vi "Apply special move.vi"(8 "error in (no error)":errorcluster, 10 "Position in":refnum<class "Position.lvclass">, 11 "DoublePush in":refnum<class "DoublePush.lvclass">) -> (0 "error out":errorcluster, 2 "Position out":refnum<class "Position.lvclass">, 3 "DoublePush out":refnum<class "DoublePush.lvclass">)   [LabVIEW 2015, in "Chesslib.lvlib" / "DoublePush.lvclass"]
uses:
  DoublePush.lvclass
  Position/Position.lvclass
  DoublePush.lvclass/DoublePush.ctl
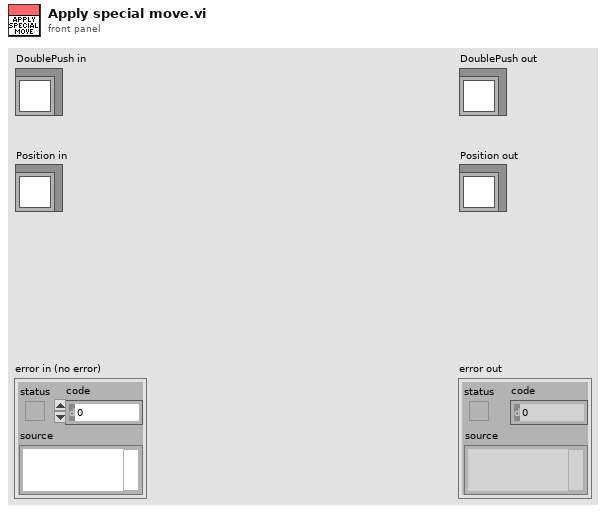
[diagram p1: front panel]
types:
  T1 = typedef "Chesslib.lvlib/Square.ctl" = cluster{"File":T2, "Rank":T3}
  T2 = typedef "Chesslib.lvlib/File.ctl" = enum8{"a", "b", "c", "d", "e", "f", "g", "h"}
  T3 = typedef "Chesslib.lvlib/Rank.ctl" = enum8{"1", "2", "3", "4", "5", "6", "7", "8"}
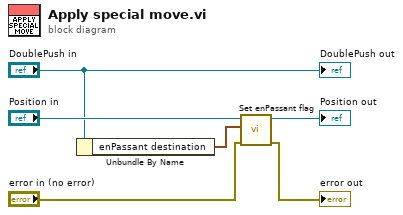
[diagram p0: block diagram]
diagram:
  n1 = Unbundle By Name("DoublePush in") -> ("enPassant destination"=w1:T1)
  n2 = call "Set enPassant flag.vi"("error in (no error)"="error in (no error)", "enPassant target"=w1, "Position in"="Position in") -> ("error out"=→"error out":errorcluster, "Position out"=→"Position out":refnum<class "Position.lvclass">)  [unwired: 7 in]
  "DoublePush out" <- "DoublePush in"
